vi "Data log.vi"(5 "COM port":refnum<visa-resource-name>="COM1", 6 "Parameter Names":string[](array[string])=["Faraday Cup Current", "Specimen Current", "Beam Dump 1 Current", "Beam Dump 2 Current"], 7 "Machine Type":u8(ring) items=["Feiss", "NVision", "Jeiss"], 8 "error in":errorcluster, 9 "milliseconds to wait":u32=1000, 10 "DataLog Files Directory":path=path "D:/3D FIB-SEM Files/FIB HV DataLog", 11 "ActiveX Container":refnum<k7>(container)) -> (0 "error out":errorcluster, 3 "reference out":refnum<k7>)   [LabVIEW 2018]
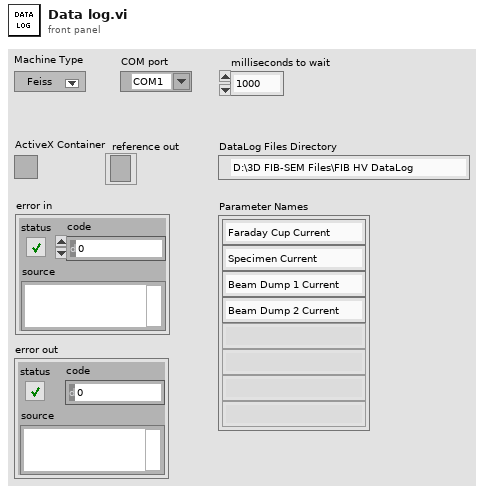
[diagram p1: front panel]
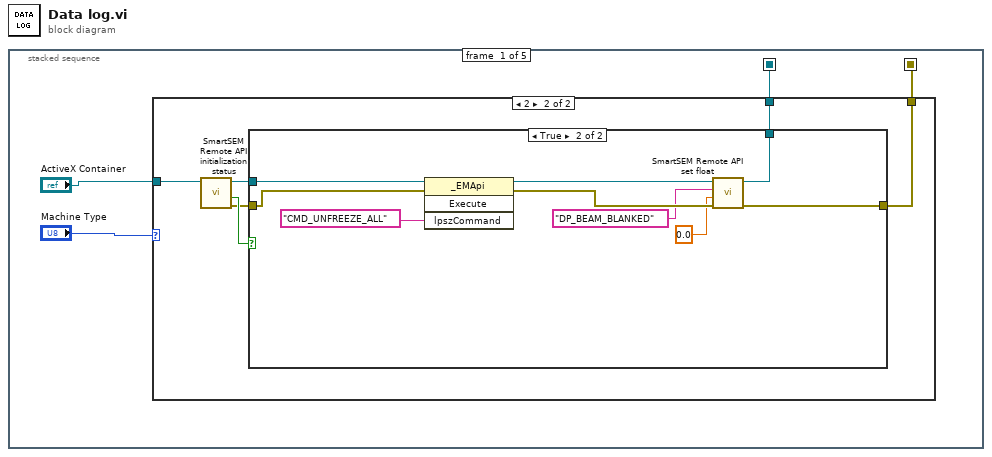
[diagram p0: block diagram]
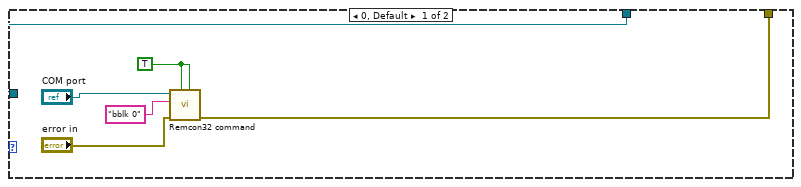
[diagram p2: hidden frame]
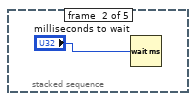
[diagram p4: hidden frame]
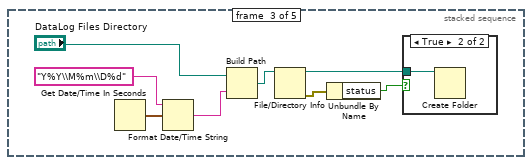
[diagram p5: hidden frame]
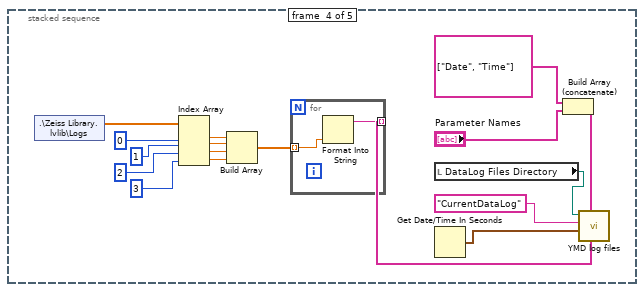
[diagram p7: hidden frame]
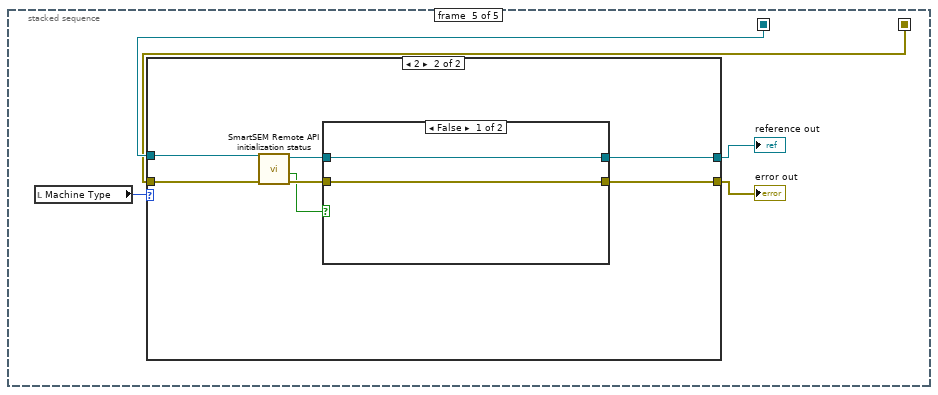
[diagram p8: hidden frame]
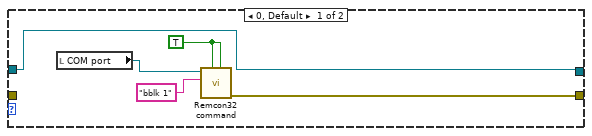
[diagram p9: hidden frame]
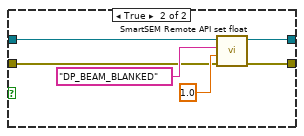
[diagram p10: hidden frame]
diagram:
  n1 = stacked-sequence {
    seq-local: [w3 _ _ _ _] -> [_ _ _ _ w60]
    seq-local: [w2 _ _ _ _] -> [_ _ _ _ w59]
    frame #0 {
      n2 = case shown="2" "Machine Type" {
        tunnel: [w6 w13] -> w2
        tunnel: [w5 w12] -> w3
        tunnel: "ActiveX Container" -> [w5 w11]
        frame 0, Default {
          w8 = TRUE ("Initialization")
          n3 = call "Remcon32 command.vi"("Close session"=w8, "Initialization"=w8, "error in"="error in", "SEM command"="bblk 0" ("write buffer"), "COM port in"="COM port") -> ("error out"=w6:errorcluster)  [unwired: 6 out]
        }
        frame 2 {
          n4 = call "SmartSEM Remote API initialization status.vi"("ActiveX Container"=w11) -> ("error out"=w14:errorcluster, "API initialized"=w16:bool, "reference out"=w15:refnum<k7>)  [unwired: 8 in]
          n5 = case shown="True" w16 {
            tunnel: w15 -> [w18 w26]
            tunnel: w14 -> [w17 w25]
            tunnel: [w17 w20] -> w13
            tunnel: [w18 w19] -> w12
            frame False {
            }
            frame True {
              n6 = invoke class="_EMApi" method="Execute"(reference=w26, error in=w25, "lpszCommand"="CMD_UNFREEZE_ALL") -> (reference out=w24:refnum<k7>, error out=w23:errorcluster)  [unwired: 1 in, 2 out]
              n7 = call "SmartSEM Remote API set float.vi"("error in"=w23, "vValue"=sgl 0.0, "lpszParam"="DP_BEAM_BLANKED", "ActiveX Container"=w24) -> ("error out"=w20:errorcluster, "reference out"=w19:refnum<k7>)  [unwired: 6 in]
            }
          }
        }
      }
    }
    frame #1 {
      n8 = Wait (ms)(milliseconds to wait="milliseconds to wait") -> ()  [unwired: 1 out]
    }
    frame #2 {
      n9 = Get Date/Time In Seconds() -> (seconds since 1Jan1904=w36:timestamp)
      n10 = Format Date/Time String(time format string (%c)="Y%Y\\M%m\\D%d", seconds (now)=w36) -> (date/time string=w32:string)  [unwired: 1 out]
      n11 = Build Path(base path="DataLog Files Directory", name or relative path=w32) -> (appended path=w30:path)
      n12 = File/Directory Info(path=w30) -> (path out=w35:path, error out=w33:errorcluster)  [unwired: 1 in, 5 out]
      n13 = Unbundle By Name(w33) -> ("status"=w34:bool)
      n14 = case shown="True" w34 {
        tunnel: w35 -> [_ w37]
        frame False {
        }
        frame True {
          n15 = Create Folder(path (use dialog)=w37) -> ()  [unwired: 1 in, 4 out]
        }
      }
    }
    frame #3 {
      n16 = shared-variable ".\\Zeiss Library.lvlib\\Logs"() -> (w46:sgl[])  [unwired: 1 in, 1 out]
      n17 = Index Array(array=w46, index #1=0 ("index"), index #2=1 ("index"), index #3=2 ("index"), index #4=3 ("index")) -> (element #1=w45:sgl, element #2=w44:sgl, element #3=w43:sgl, element #4=w42:sgl)
      n18 = Build Array(w45, w44, w43, w42) -> (w54:sgl[])
      n19 = for {
        tunnel: w54 -> [w55] mode=indexing
        tunnel: [w56] -> w47 mode=indexing
        n20 = Format Into String(w55) -> (resulting string=w56:string)  [unwired: 3 in, 1 out]
      }
      n21 = local read "DataLog Files Directory"() -> (w52:path)
      n22 = Get Date/Time In Seconds() -> (seconds since 1Jan1904=w53:timestamp)
      n23 = Build Array (concatenate)(string[] ["Date", "Time"] ("Parameter Names"), "Parameter Names") -> (w48:string[])
      n24 = call "YMD log files.vi"("Input text array"=w47, "Input header array"=w48, "current time"=w53, "Log file name"="CurrentDataLog" ("string"), "Log file path"=w52) -> ()  [unwired: 7 in]
    }
    frame #4 {
      n25 = local read "Machine Type"() -> (w61:u8)
      n26 = case shown="2" w61 {
        tunnel: w60 -> [w62 w70]
        tunnel: w59 -> [_ w69]
        tunnel: [w63 w68] -> w57
        tunnel: [w62 w67] -> w58
        frame 0, Default {
          w65 = TRUE ("Initialization")
          n27 = local read "COM port"() -> (w64:refnum<visa-resource-name>)
          n28 = call "Remcon32 command.vi"("Close session"=w65, "Initialization"=w65, "SEM command"="bblk 1" ("write buffer"), "COM port in"=w64) -> ("error out"=w63:errorcluster)  [unwired: 1 in, 6 out]
        }
        frame 2 {
          n29 = call "SmartSEM Remote API initialization status.vi"("error in"=w69, "ActiveX Container"=w70) -> ("error out"=w72:errorcluster, "API initialized"=w71:bool, "reference out"=w73:refnum<k7>)  [unwired: 7 in]
          n30 = case shown="False" w71 {
            tunnel: w73 -> [w75 w79]
            tunnel: w72 -> [w74 w78]
            tunnel: [w74 w77] -> w68
            tunnel: [w75 w76] -> w67
            frame False {
            }
            frame True {
              n31 = call "SmartSEM Remote API set float.vi"("error in"=w78, "vValue"=sgl 1.0, "lpszParam"="DP_BEAM_BLANKED", "ActiveX Container"=w79) -> ("error out"=w77:errorcluster, "reference out"=w76:refnum<k7>)  [unwired: 6 in]
            }
          }
        }
      }
      "error out" <- w57
      "reference out" <- w58
    }
  }
